vi "Status - motion with X and Y.vi"(8 "error in (no error)":errorcluster, 11 "VISA resource name":refnum<visa-resource-name>) -> (0 "error out":errorcluster, 1 "Positions, counts":i32[](array[numeric]), 3 "VISA resource out":refnum<visa-resource-name>, 4 "Motion Stopped":bool, 5 "Limit Switch Activated":bool)   [LabVIEW 2017]
doc: "Read X and Y during motion.\nAlso detect two VXM control characters, \n^ end of motion and \nO, limit switch"
panel:
  out "i":i32
  # "Won't read\nall four while in motion,\nonly two !!!\nManual page 13\n\nwon't read Z and T while \nX or Z is in motion"
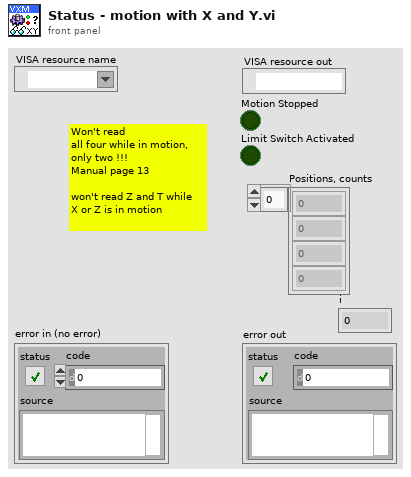
[diagram p1: front panel]
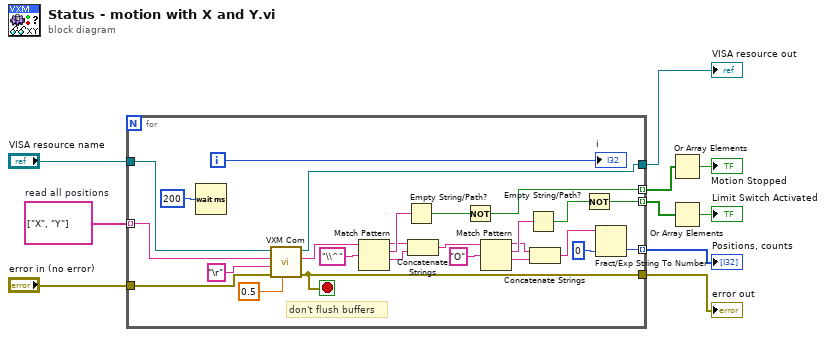
[diagram p0: block diagram]
diagram:
  w1 = string[] ["X", "Y"]  # read all positions
  n1 = for {
    tunnel: [w34] -> w6 mode=indexing
    tunnel: w1 -> [w33] mode=indexing
    tunnel: "VISA resource name" -> [w32]
    tunnel: [w31] -> w9
    tunnel: [w29] -> w8
    tunnel: "error in (no error)" -> [w30]
    tunnel: [w25] -> w5 mode=indexing
    tunnel: [w15] -> w4 mode=indexing
    i -> [w11]
    stop <- w29 stop-if-true
    # "don't flush buffers"
    n2 = Wait (ms)(milliseconds to wait=u32 200) -> ()  [unwired: 1 out]
    n3 = call "VXM Com.vi"("Timeout, s"=0.5, "error in (no error)"=w30, "Termination String ('/' codes)"="\r", "Write Buffer ('/' codes)"=w33, "VISA resource name"=w32) -> ("error out"=w29:errorcluster, "Response String ('/' codes)"=w14:string, "VISA resource out"=w31:refnum<visa-resource-name>)  [unwired: 4 in]
    n4 = Match Pattern(string=w14, regular expression="\\^") -> (before substring=w24:string, match substring=w27:string, after substring=w23:string)  [unwired: 1 in, 1 out]
    n5 = Empty String/Path?(string/path=w27) -> (empty?=w26:bool)
    n6 = Concatenate Strings(w24, w23) -> (w19:string)
    n7 = Not(x=w26) -> (.not. x?=w25:bool)
    n8 = Match Pattern(string=w19, regular expression="O") -> (before substring=w18:string, match substring=w21:string, after substring=w17:string)  [unwired: 1 in, 1 out]
    n9 = Empty String/Path?(string/path=w21) -> (empty?=w22:bool)
    n10 = Concatenate Strings(w18, w17) -> (w16:string)
    n11 = Not(x=w22) -> (.not. x?=w15:bool)
    n12 = Fract/Exp String To Number(string=w16, default (0 dbl)=0 ("default (0 DBL)")) -> (number=w34:i32)  [unwired: 2 in, 1 out]
    "i" <- w11
  }
  "VISA resource out" <- w9
  "error out" <- w8
  "Positions, counts" <- w6
  n13 = Or Array Elements(Boolean array=w5) -> (logical OR=→"Motion Stopped":bool)
  n14 = Or Array Elements(Boolean array=w4) -> (logical OR=→"Limit Switch Activated":bool)
